vi "Find Workspace.vi"(6 "Pickup_Test_Number":dbl, 8 "error in (no error)":errorcluster, 9 "Assembly Type":string, 10 "Control In":T2={"I-O.lvclass"=refnum, "Gantry"=refnum, "Dispenser"="COM1"}, 11 "Component.lvclass":refnum<class "Component Tray.lvclass">) -> (0 "error out":errorcluster, 1 "Workspace":T1, 2 "Control Out":T2={"I-O.lvclass"=refnum, "Gantry"=refnum, "Dispenser"="COM1"}, 3 "Workspace Out":refnum<class "Component Tray.lvclass">)   [LabVIEW 2021, in "Component Tray.lvclass"]
uses:
  Component Tray.lvclass
  Controller/Controllers.ctl
  Controller/I-O/I-O.lvclass
  C:/Program Files (x86)/Aerotech/A3200/LabVIEW/2010/Bin/Aerotech.A3200.dll
  Program Files (x86)/Aerotech/A3200/LabVIEW/2010/Bin/Aerotech.A3200.dll
  Workspace.ctl
  C:/Users/HEP/Documents/GitHub/Gantry/UCSB-Gantry-HEP-main/Classes/Workspace/Fixture.lvclass
  Fixture.lvclass/Fixture.ctl
  Component Tray.lvclass/Component Tray.ctl
  Read Fixture ID.vi
  Read Position.vi
  Fixture.lvclass
  Controller/Controller.lvclass
panel:
  out "XYZTheta":dbl[](array[numeric]) format="%#.6g"
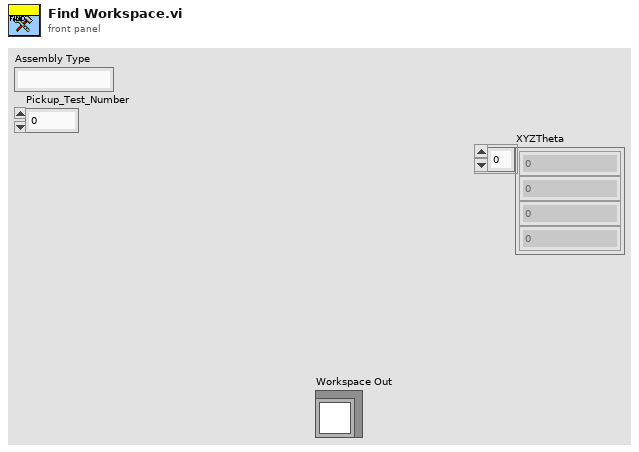
[diagram p1: front panel]
types:
  T1 = typedef "Fixture.lvclass/Workspace.ctl" = cluster{"XYZTheta":dbl[], "Workspace Valve":i32, "Workspace Sensor":i32}
  T2 = typedef "Controller.lvclass/Controllers.ctl" = cluster{"I-O.lvclass":refnum<class "I-O.lvclass">, "Gantry":refnum<k24>, "Dispenser":refnum<visa-resource-name>}
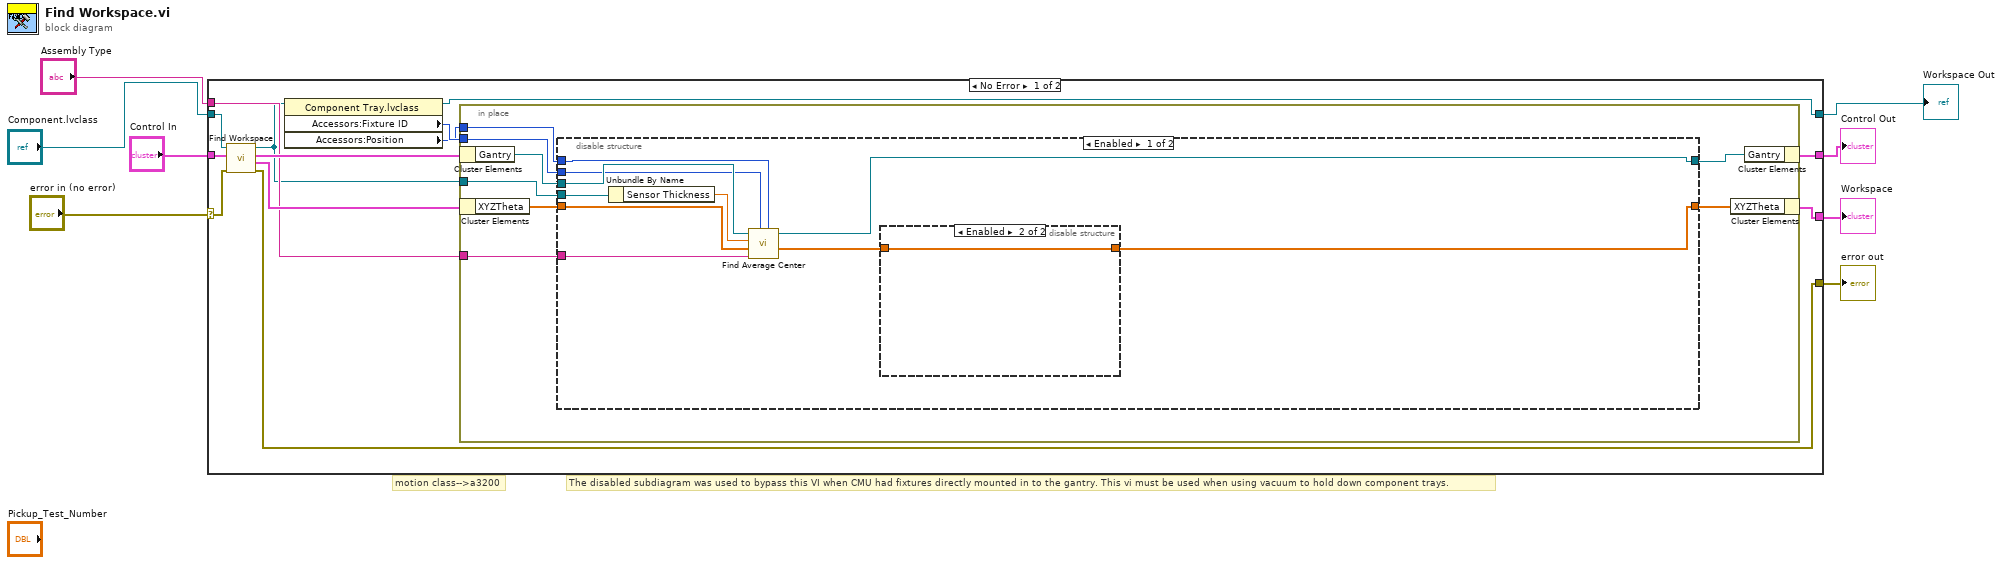
[diagram p0: block diagram]
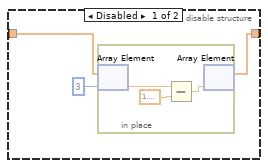
[diagram p2: hidden frame]
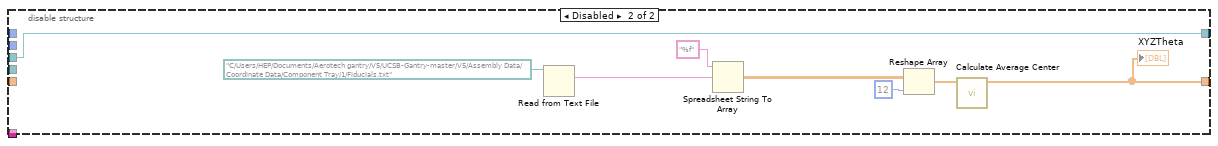
[diagram p3: hidden frame]
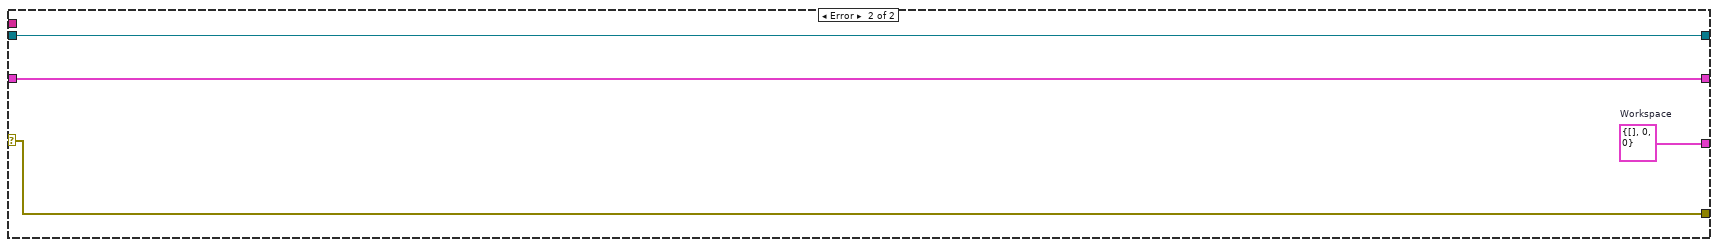
[diagram p4: hidden frame]
diagram:
  # "The disabled subdiagram was used to bypass this VI when CMU had fixtures directly mounted in to the gantry. This vi must be used when using vacuum to hold down component trays."
  # "motion class-->a3200"
  n1 = case shown="No Error" "error in (no error)" {
    selector: "error in (no error)" -> [w19 w58]
    tunnel: [w15 w57] -> w8
    tunnel: [w21 w58] -> w7
    tunnel: [w14 w56] -> w6
    tunnel: "Control In" -> [w18 w57]
    tunnel: [w12 w55] -> w3
    tunnel: "Component.lvclass" -> [w17 w55]
    tunnel: "Assembly Type" -> [w11 _]
    frame No Error {
      n2 = call-parent "Find Workspace.vi"("Error In"=w19, "Control In"=w18, "Workspace In"=w17) -> ("Error Out"=w21:errorcluster, 1:"Workspace Out"=w20:T1, "Control Out"=w16:T2, 3:"Workspace Out"=w9:refnum<class "Component Tray.lvclass">)  [unwired: 5 in]
      n3 = property class="Component Tray.lvclass"(reference=w9) -> (reference out=w12:refnum<class "Component Tray.lvclass">, "Accessors:Fixture ID"=w13:i32, "Accessors:Position"=w10:i32)  [unwired: 1 in, 1 out]
      n4 = in-place {
        in-place-border: w13 -> [w28]
        in-place-border: w10 -> [w29]
        in-place-border: w11 -> [w23]
        in-place-border: w9 -> [w22]
        n5 = in-place-cluster #1(w16) -> ("Gantry"=w27:refnum<k24>)
        n6 = in-place-cluster #2(w20) -> ("XYZTheta"=w26:dbl[])
        n7 = disable-structure shown="Enabled" {
          disable-tunnel: w29 -> [w36 _]
          disable-tunnel: w28 -> [w35 _]
          disable-tunnel: w27 -> [w39 w47]
          disable-tunnel: w26 -> [w38 _]
          disable-tunnel: [w33 w48] -> w25
          disable-tunnel: [w37 w47] -> w24
          disable-tunnel: w23 -> [w32 _]
          disable-tunnel: w22 -> [w31 _]
          frame Enabled {
            n8 = Unbundle By Name(w31) -> ("Sensor Thickness"=w30:dbl)
            n9 = call "Find Average Center.vi"("Position"=w36, "Tray Number"=w35, "Assembly Type"=w32, "XYZTheta"=w38, "Sensor Thickness"=w30, "Gantry In"=w39) -> ("XYZTheta"=w34:dbl[], "Gantry Out"=w37:refnum<k24>)  [unwired: 4 in]
            n10 = disable-structure shown="Enabled" {
              disable-tunnel: w34 -> [w42 w46]
              disable-tunnel: [w40 w46] -> w33
              frame Disabled {
                n11 = in-place {
                  n12 = in-place-array #3(w42, 3) -> (w45:dbl)
                  n13 = Subtract(x=w45, y=1.5707963267948966) -> (x-y=w43:dbl)
                  n14 = in-place-array #3(w43) -> (w40:dbl[])  [unwired: 1 out]
                }
              }
              frame Enabled {
              }
            }
          }
          frame Disabled {
            n15 = Read from Text File(file (use dialog)=path "C:/Users/HEP/Documents/Aerotech gantry/V5/UCSB-Gantry-master/V5/Assembly Data/Coordinate Data/Component Tray/1/Fiducials.txt") -> (text=w52:string)  [unwired: 3 in, 3 out]
            n16 = Spreadsheet String To Array(format string="%f", spreadsheet string=w52) -> (array=w51:dbl[][])  [unwired: 2 in]
            n17 = Reshape Array(w51, 12 ("dimension size")) -> (w49:dbl[])
            n18 = call "Calculate Average Center.vi"("Gantry Fiducials"=w49) -> ("XYZTheta"=w48:dbl[])  [unwired: 8 in, 2 out]
            "XYZTheta" <- w48
          }
        }
        n19 = in-place-cluster #2("XYZTheta"=w25) -> (w14:T1)
        n20 = in-place-cluster #1("Gantry"=w24) -> (w15:T2)
      }
    }
    frame Error {
      w56 = T1 {"XYZTheta"=[], "Workspace Valve"=0, "Workspace Sensor"=0}  # Workspace
    }
  }
  "error out" <- w7
  "Control Out" <- w8
  "Workspace" <- w6
  "Workspace Out" <- w3
